vi "Restore Session Defaults.vi"(0 "Session Handle":T1, 11 "error in (no error)":errorcluster) -> (4 "Session Handle out":T1, 15 "error out":errorcluster)   [LabVIEW 2019, in "HTS.lvlib" / "Engine.lvclass"]
doc: "Restores session defaults"
uses:
  Engine.lvclass
  Program Files (x86)/National Instruments/LabVIEW 2020/user.lib/_Session Fwk/Session - Root.lvclass
  Typedefs/Session Handle.ctl
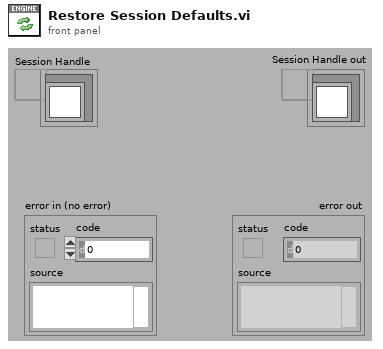
[diagram p1: front panel]
types:
  T1 = typedef "HTS.lvlib/Engine.lvclass/Session Handle.ctl" = refnum<data-value>
  T2 = typedef "Session - Root.lvclass/Session Handle.ctl" = refnum<data-value>
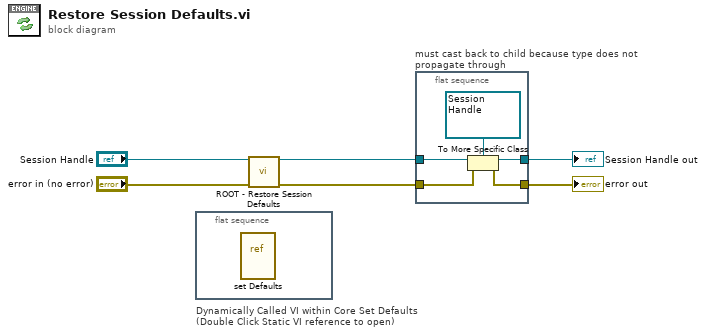
[diagram p0: block diagram]
diagram:
  n1 = flat-sequence "Dynamically Called VI within Core Set Defaults\n(Double Click Static VI reference to open)" {
    frame #0 {
      n2 = vi-ref "set Defaults.vi"() -> ()  [unwired: 1 out]
    }
  }
  n3 = call "ROOT - Restore Session Defaults.vi"("Session Handle in"="Session Handle", "error in (no error)"="error in (no error)") -> ("Session Handle out"=w5:T2, "error out"=w3:errorcluster)  [unwired: 12 in]
  n4 = flat-sequence "must cast back to child because type does not propagate through" {
    tunnel: w5 -> [w11]
    tunnel: w3 -> [w10]
    tunnel: [w9] -> w2
    tunnel: [w8] -> w1
    frame #0 {
      n5 = To More Specific Class(target class=T1 refnum ("Session Handle"), reference=w11, error in=w10) -> (specific class reference=w8:T1, error out=w9:errorcluster)
    }
  }
  "error out" <- w2
  "Session Handle out" <- w1
